vi "215.Zpos (SubVI).vi"(8 "error in (no error)":errorcluster, 9 "Z":i32=1200 min=0 max=1200 step=1, 11 "VISA resource name":refnum<visa-resource-name>="COM7") -> (0 "error out":errorcluster, 1 "Receive string":string, 2 "Connected":bool, 3 "VISA Out":refnum<visa-resource-name>)   [LabVIEW 2020]
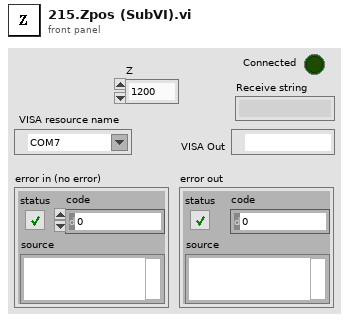
[diagram p1: front panel]
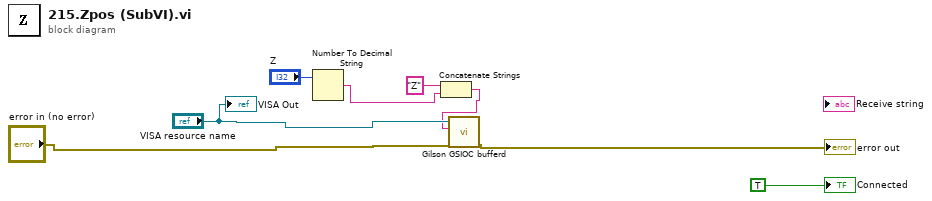
[diagram p0: block diagram]
diagram:
  n1 = Number To Decimal String(number="Z") -> (decimal integer string=w7:string)  [unwired: 1 in]
  n2 = Concatenate Strings("Z" ("string"), w7) -> (w2:string)
  n3 = call <instrlib>:"Gilson GSIOC bufferd.vi"("error in (no error)"="error in (no error)", "Bufferd command"=w2, "VISA resource name"="VISA resource name") -> ("error out"=→"error out":errorcluster)  [unwired: 6 in, 2 out]
  "Connected" <- TRUE
  "VISA Out" <- "VISA resource name"
